vi "Create (Dimensions).vi"(8 "error in (no error)":errorcluster, 10 "Dimensions":i32[](array[numeric]), 11 "DBL array in":dbl[](array[numeric])) -> (0 "error out":errorcluster, 3 "Float64Array out":refnum<class "Float64Array.lvclass">)   [LabVIEW 2013, in "MDSplus.lvlib" / "Float64Array.lvclass"]
uses:
  <vilib>/MDSplus/Classes/Data_Class/Array_Class/Float64Array_Class/Float64Array.lvclass
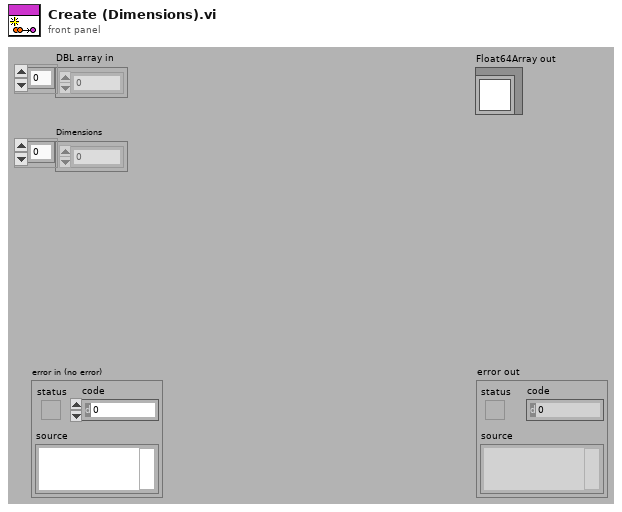
[diagram p1: front panel]
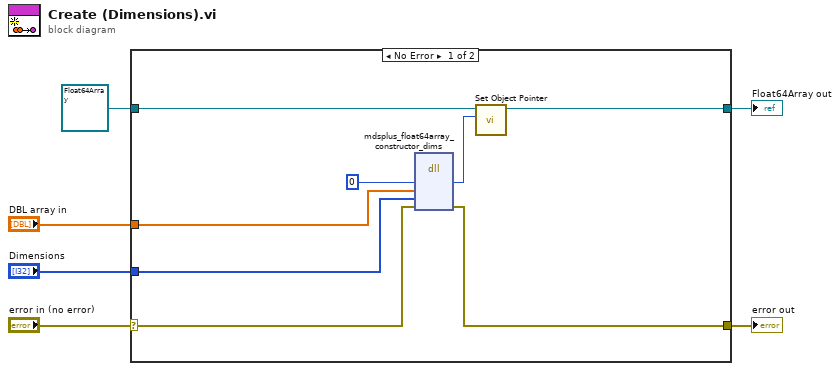
[diagram p0: block diagram]
diagram:
  n1 = case shown="No Error" "error in (no error)" {
    selector: "error in (no error)" -> [w12 w16]
    tunnel: [w7 w16] -> w5
    tunnel: [w10 w15] -> w3
    tunnel: refnum<class "Float64Array.lvclass"> refnum ("Float32 in") -> [w11 w15]
    tunnel: "DBL array in" -> [w9 _]
    tunnel: "Dimensions" -> [w8 _]
    frame No Error {
      n2 = dll-call lib="MDSobjectsLVShr" fn="mdsplus_float64array_constructor_dims"("lvFloat64ArrayPtrOut"=i64 0 ("lvTreePtr"), "lvDblArrHdlIn"=w9, "lvIntArrHdlIn"=w8, "error"=w12) -> ("lvFloat64ArrayPtrOut"=w13:i64, "error"=w7:errorcluster)  [unwired: 6 in, 2 out]
      n3 = call-dynamic "Set Object Pointer.vi"("Object Pointer"=w13, "Data in"=w11) -> ("Data out"=w10:refnum<class "Float64Array.lvclass">)  [unwired: 9 in]
    }
    frame Error {
    }
  }
  "error out" <- w5
  "Float64Array out" <- w3
